vi "ResultsDB Create Barcode Items.vi"(6 "Order":T2, 8 "error in (no error)":errorcluster, 9 "File format":T1=".tdms", 10 "StationName":string, 11 "MainBarcode":string) -> (0 "error out":errorcluster, 2 "ResultFilePath":path, 3 "Row Numbers":string)   [LabVIEW 2021, in "SQLite.lvclass"]
doc: "开始测试时根据条目自动创建条目条目，生产文件路径。\n#2020-6-8 13:25:45"
uses:
  SQLite.lvclass
  Order.ctl
  File Format.ctl
  <vilib>/Utility/error.llb/Trim Whitespace.vi
  SQLite.lvclass/SQLite.ctl
  <userlib>/LabSQL/LabSQL.lvlib
  <userlib>/sushu/sushu.lvlib
  vi.lib_New/TopPath/TopPath.lvlib
panel:
  in  "error in (no error) 2":errorcluster
  out "CMD":string
  out "error out 2":errorcluster
  out "source":string
  out "match substring":string
  out "number (0 to 1)":dbl
  # "SQLITE_CONSTRAINT: UNIQUE constraint failed"
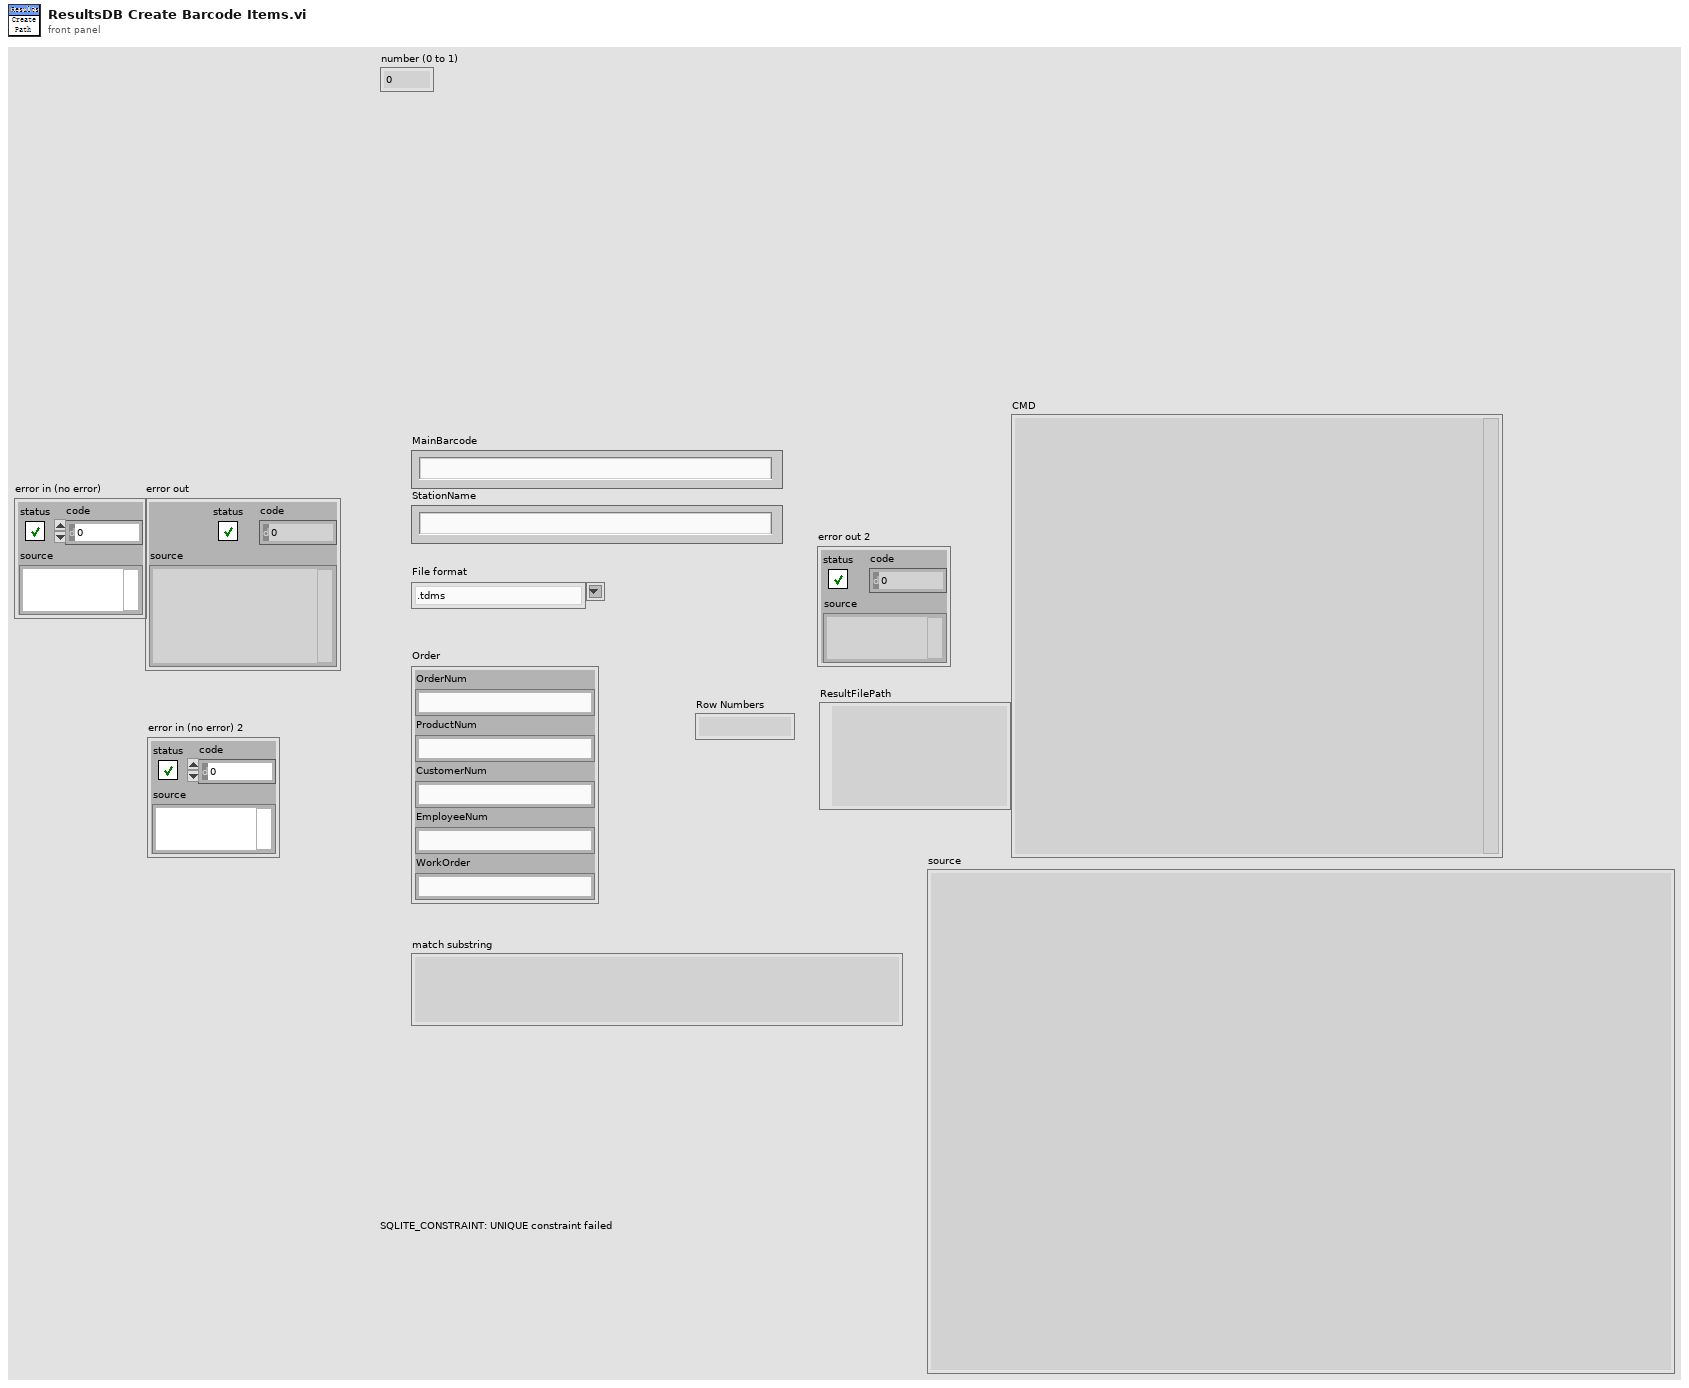
[diagram p1: front panel]
types:
  T1 = typedef "SQLite.lvclass/File Format.ctl" = string
  T2 = typedef "SQLite.lvclass/Order.ctl" = cluster{"OrderNum":string, "ProductNum":string, "CustomerNum":string, "EmployeeNum":string, "WorkOrder":string}
  T3 = cluster{"Core":cluster{"Current VI Reference":refnum<vi>, "Close Panel on Exit?":bool}, "VI Name":string, "Row Numbers":string, "Update?":bool, "Results Folder path":path, "CMD":string, "RowNum":i32, "ResultFilePath":path, "InsertTimes":i32}
  T4 = enum16{"Other", "SQL2008", "SQLite", "Access", "MySQL"}
  T5 = typedef "TopPath.lvlib/Top Path.ctl" = cluster{"LV Source":path, "FilePath":path, "Data":path}
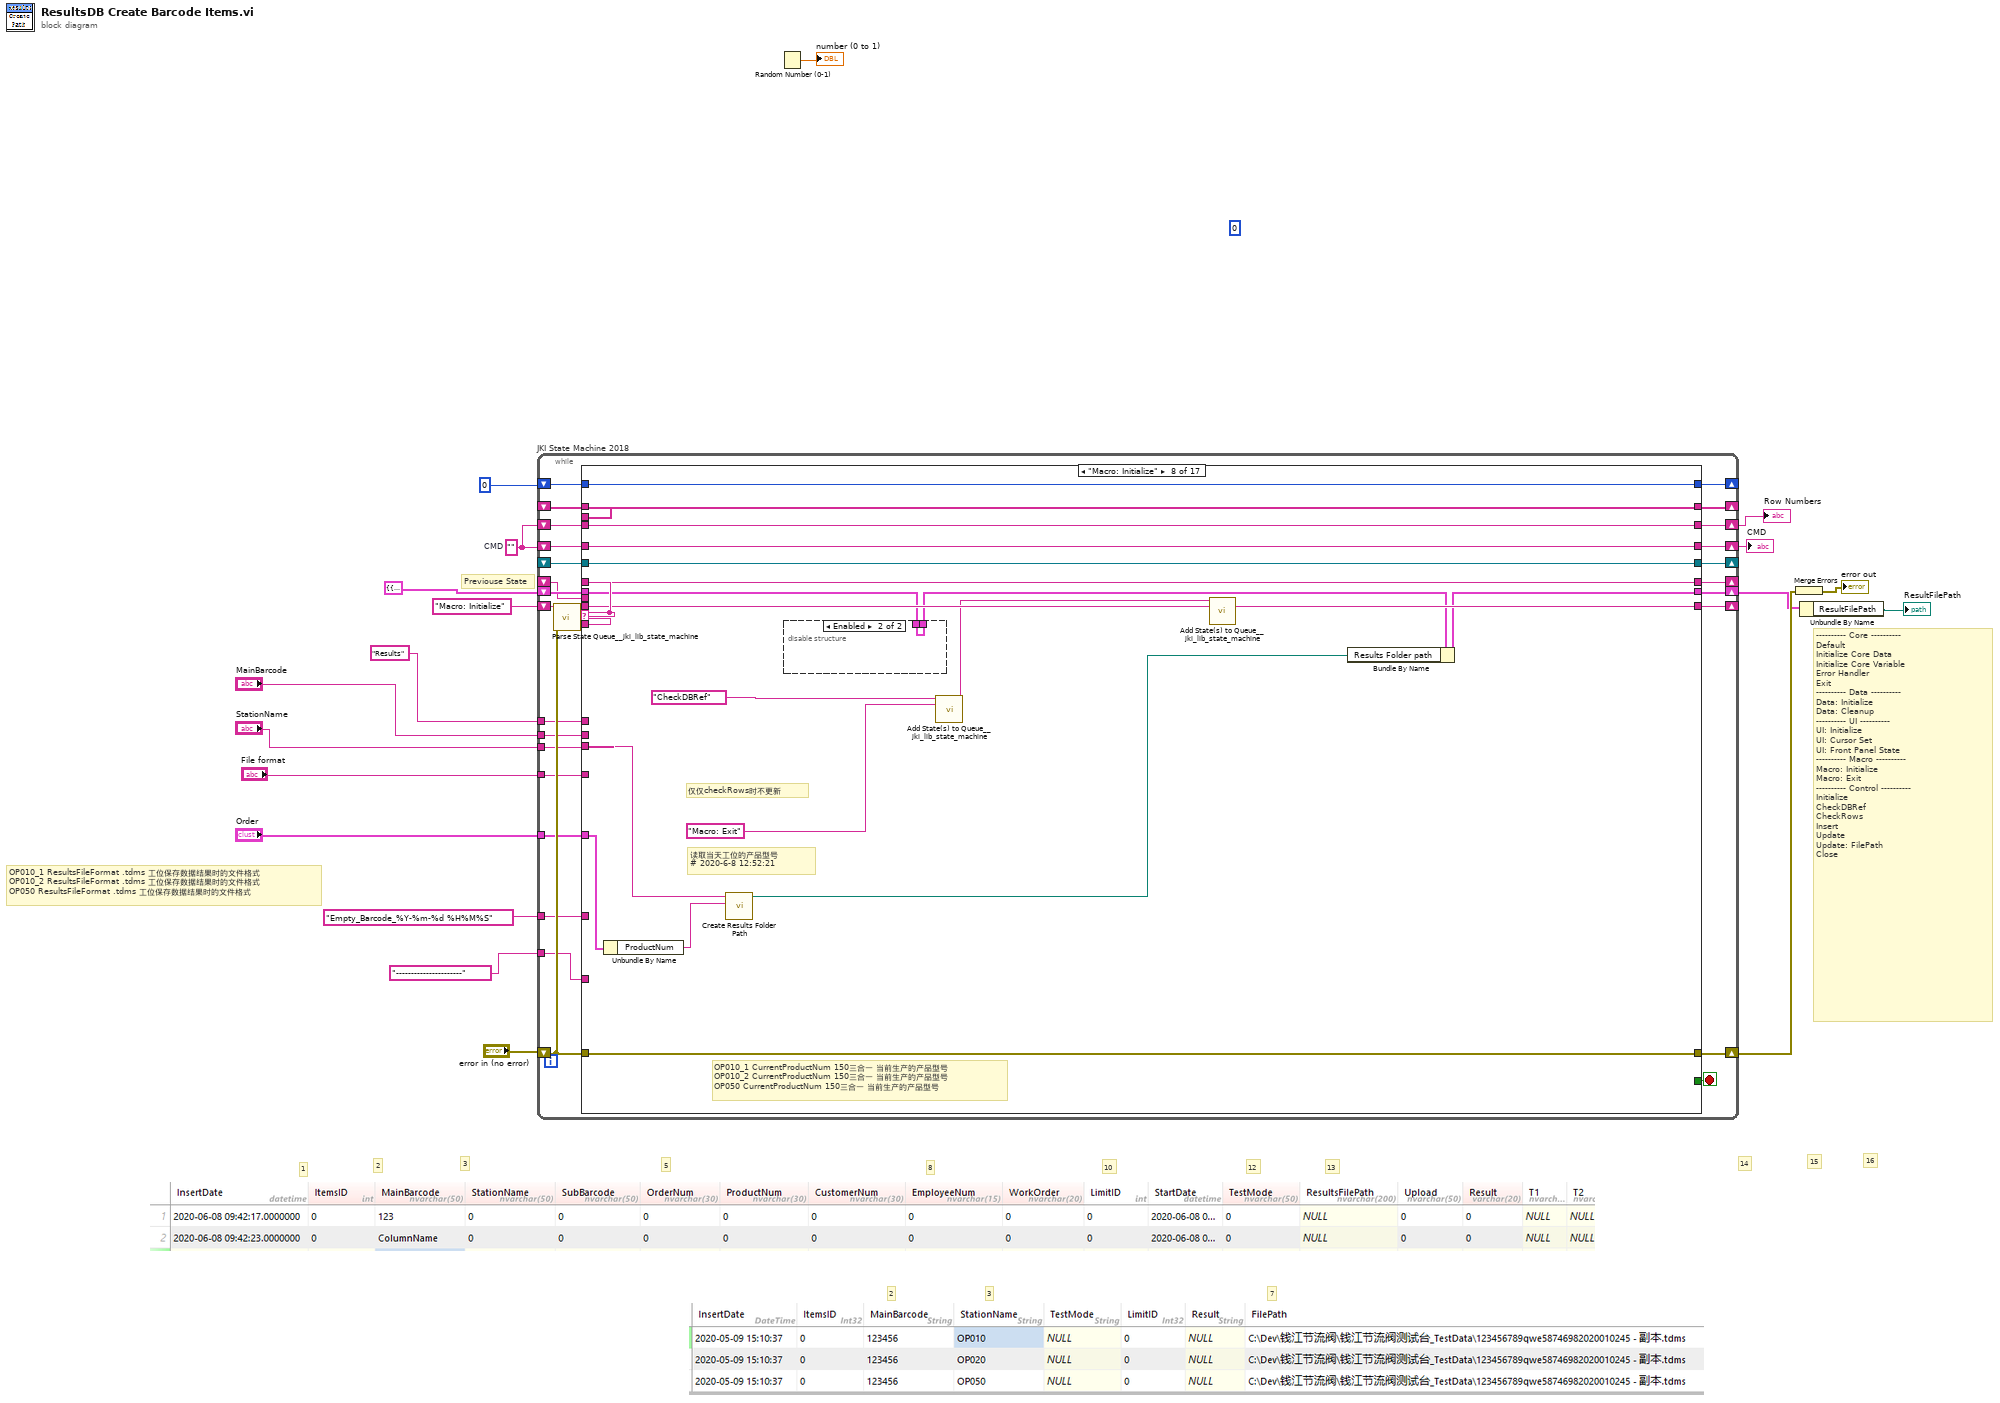
[diagram p0: block diagram]
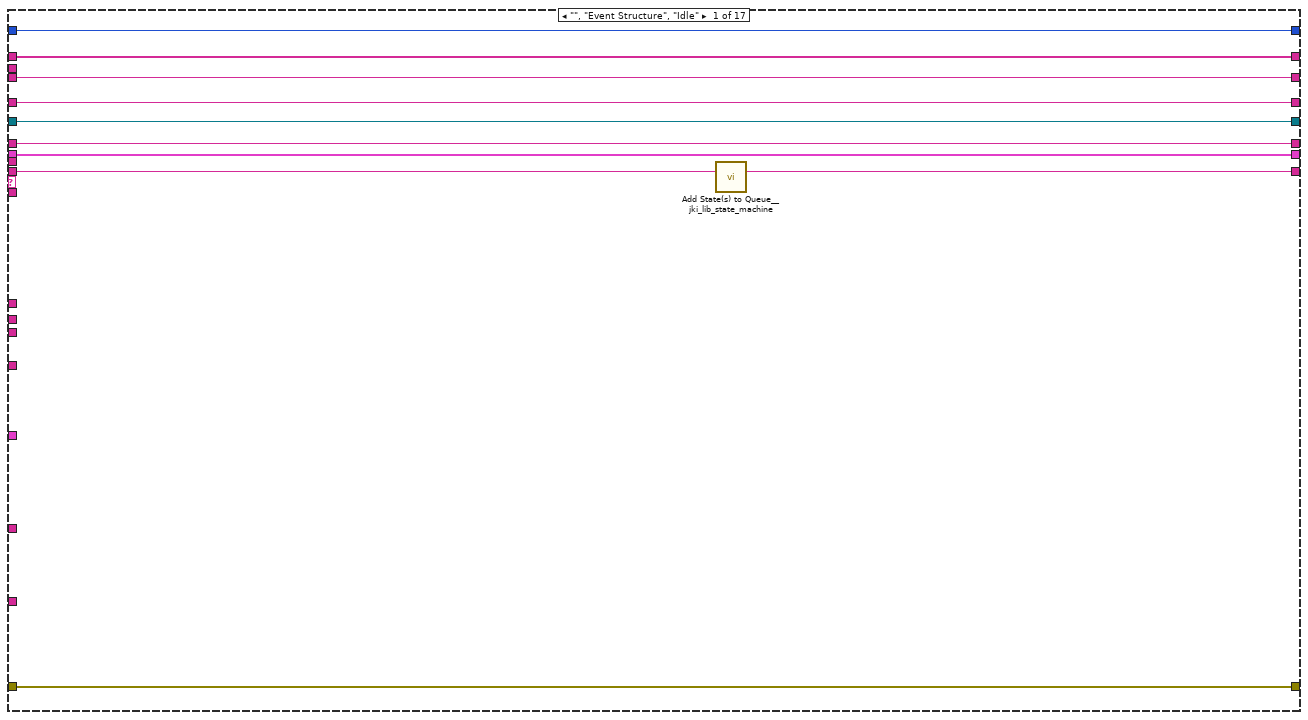
[diagram p2: hidden frame]
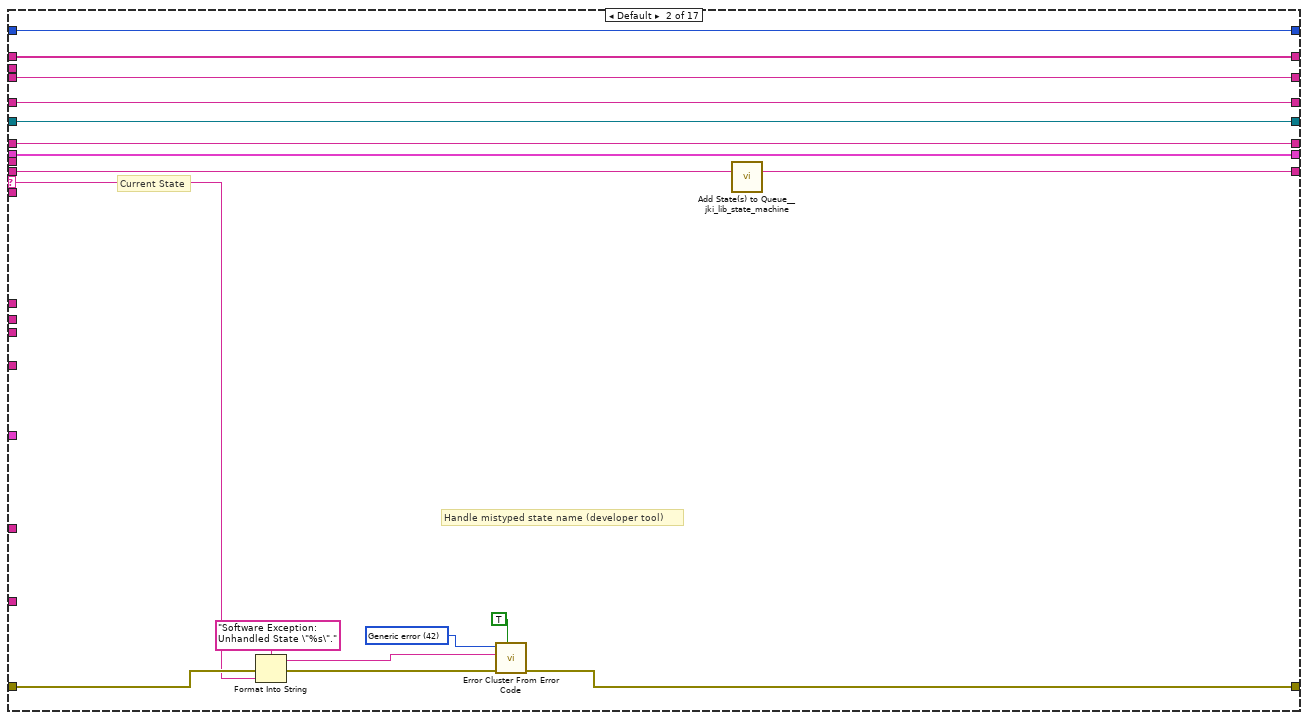
[diagram p3: hidden frame]
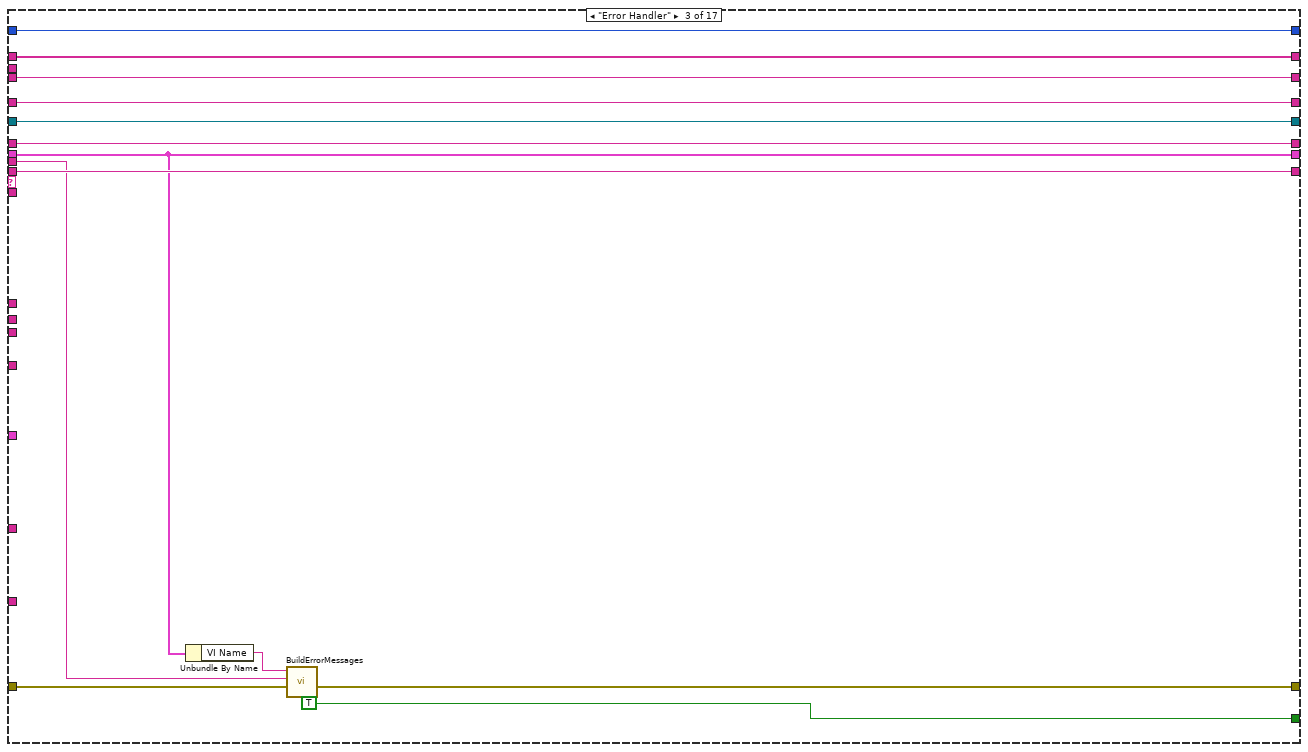
[diagram p4: hidden frame]
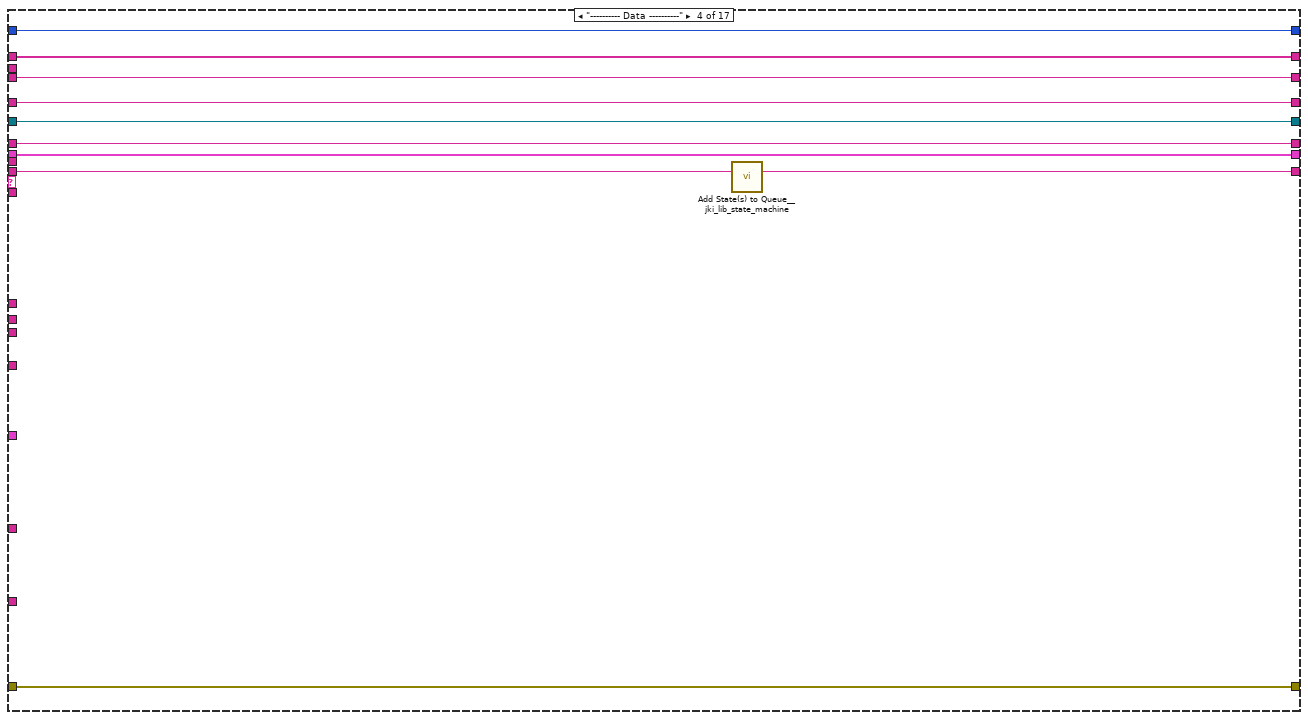
[diagram p5: hidden frame]
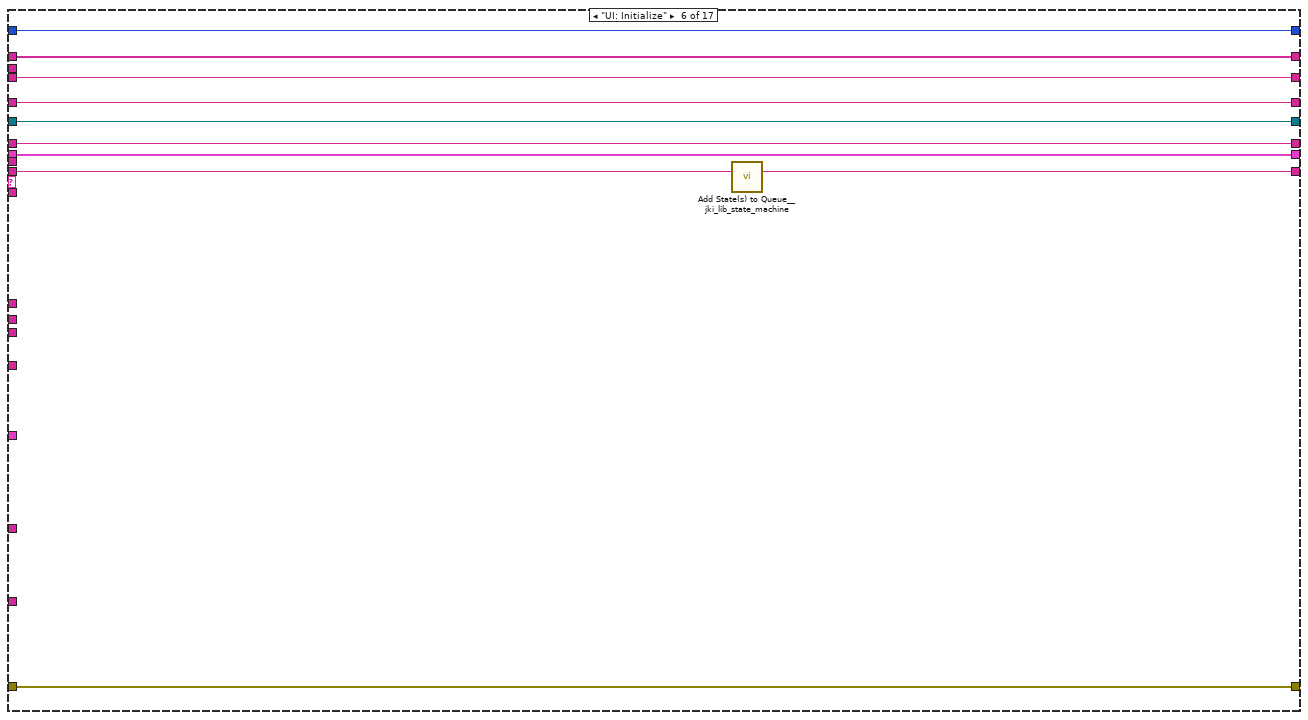
[diagram p7: hidden frame]
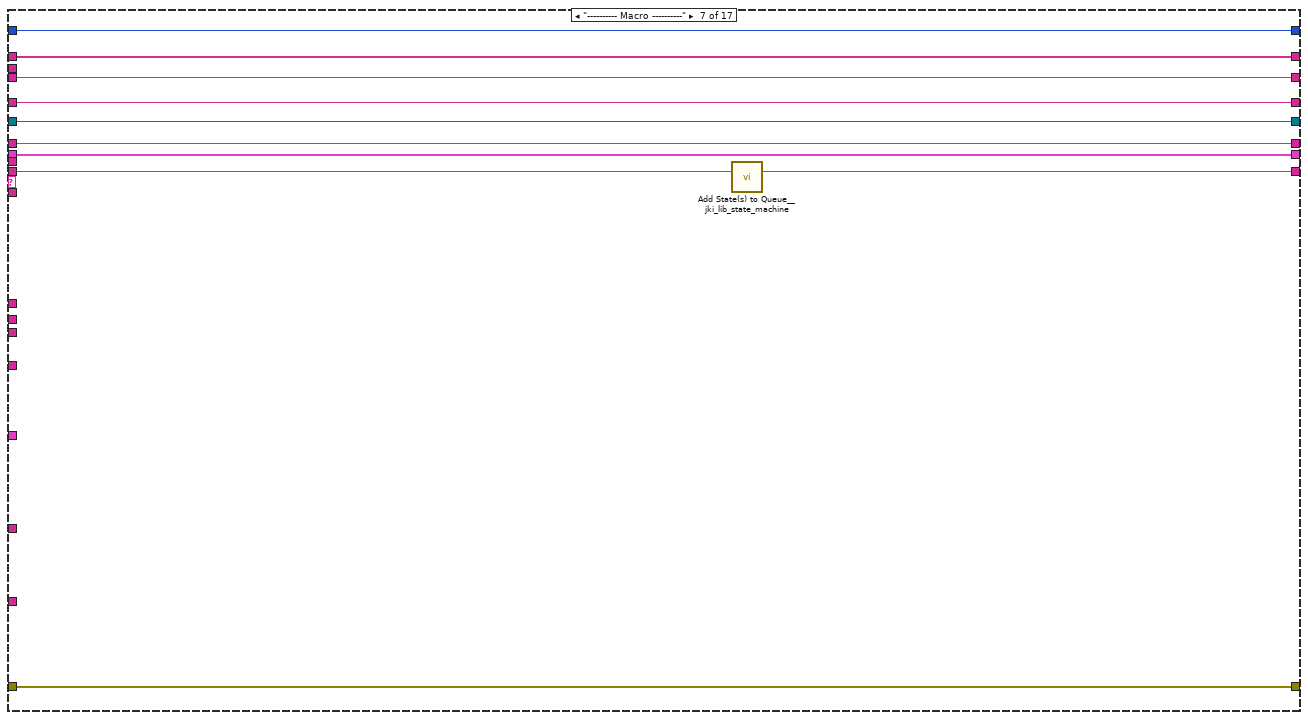
[diagram p8: hidden frame]
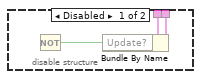
[diagram p9: hidden frame]
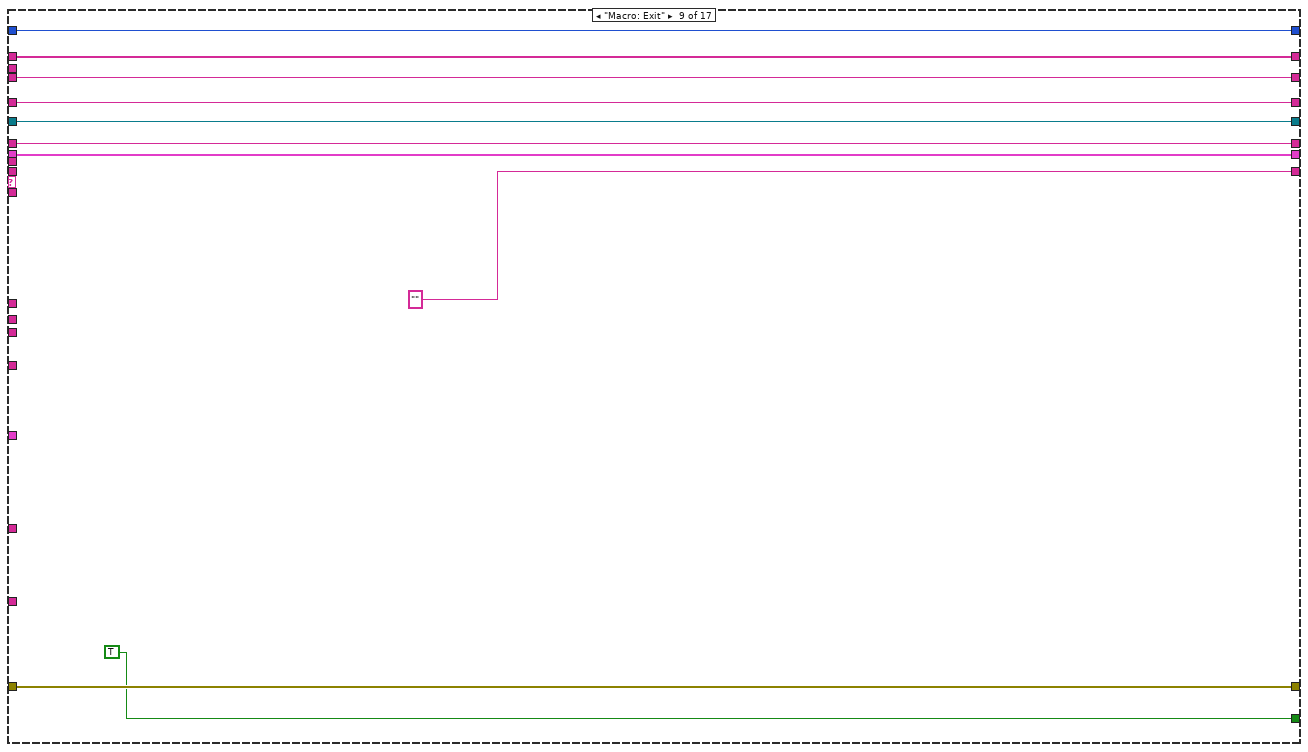
[diagram p10: hidden frame]
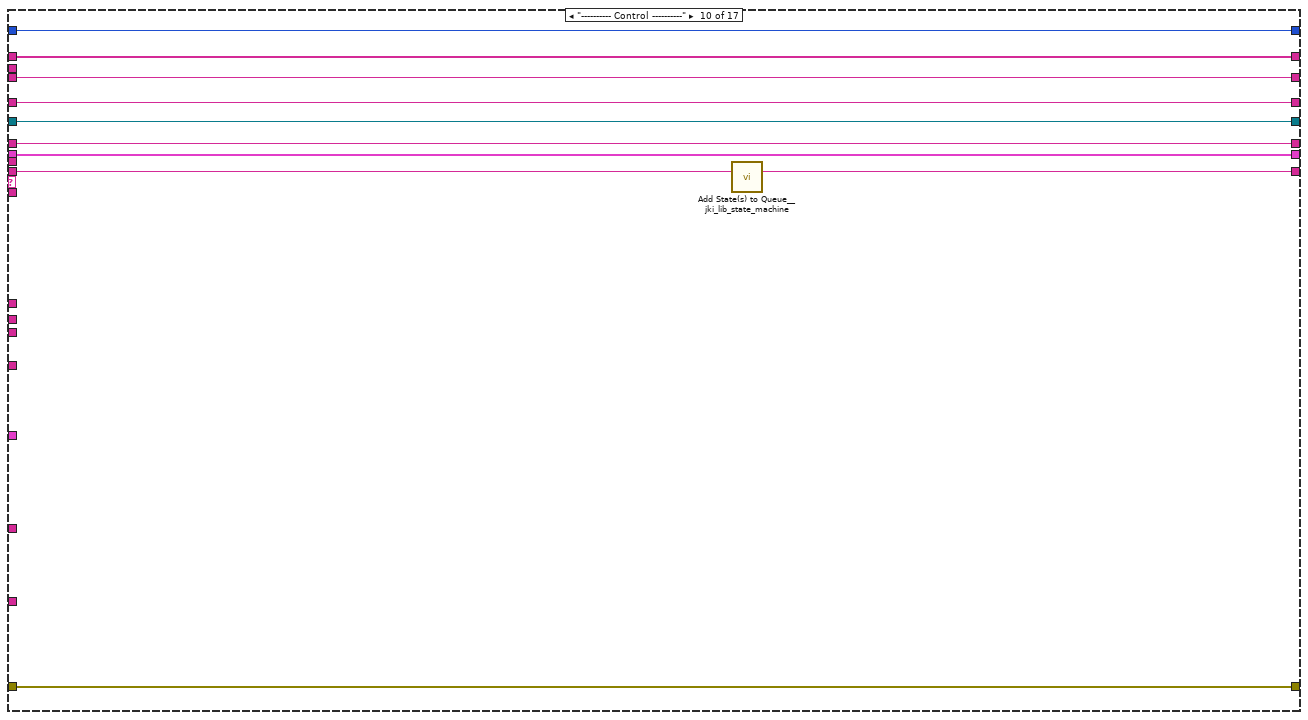
[diagram p11: hidden frame]
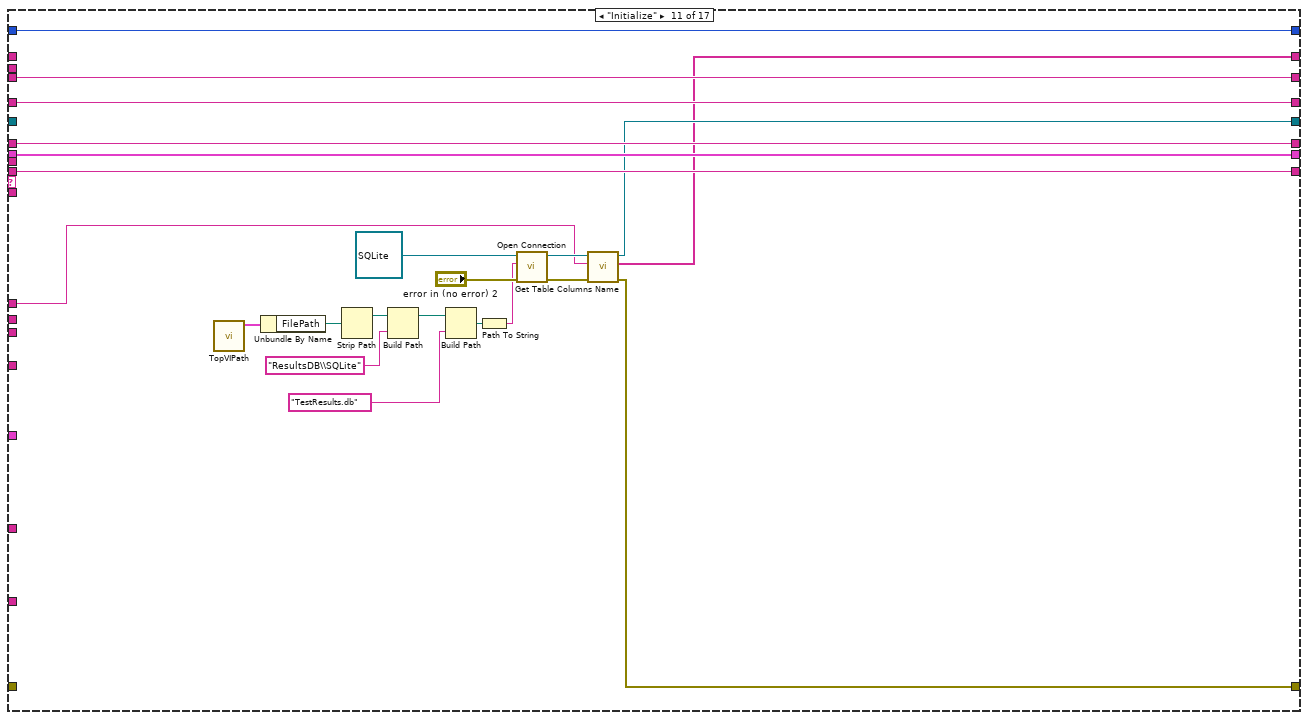
[diagram p12: hidden frame]
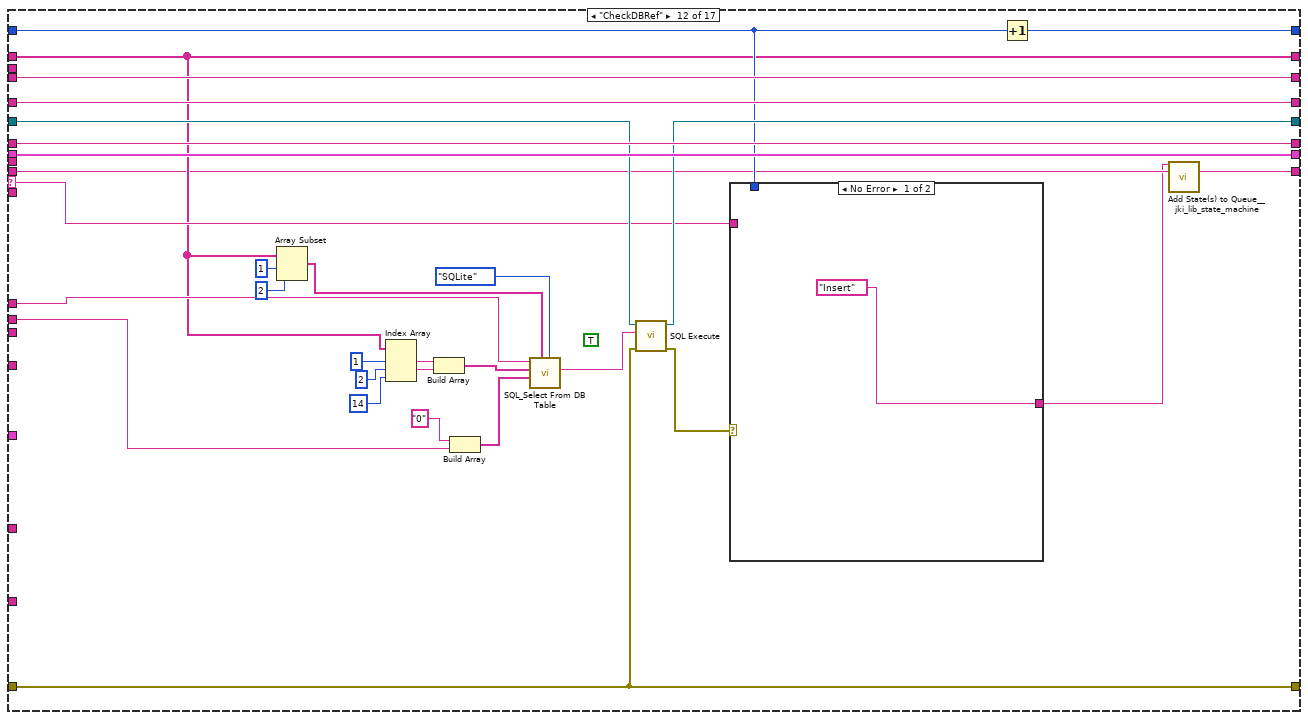
[diagram p13: hidden frame]
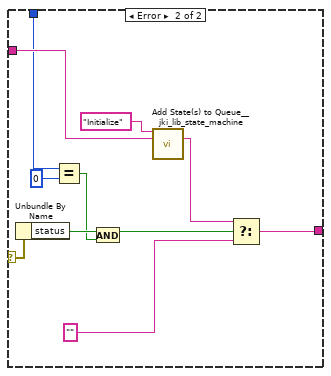
[diagram p14: hidden frame]
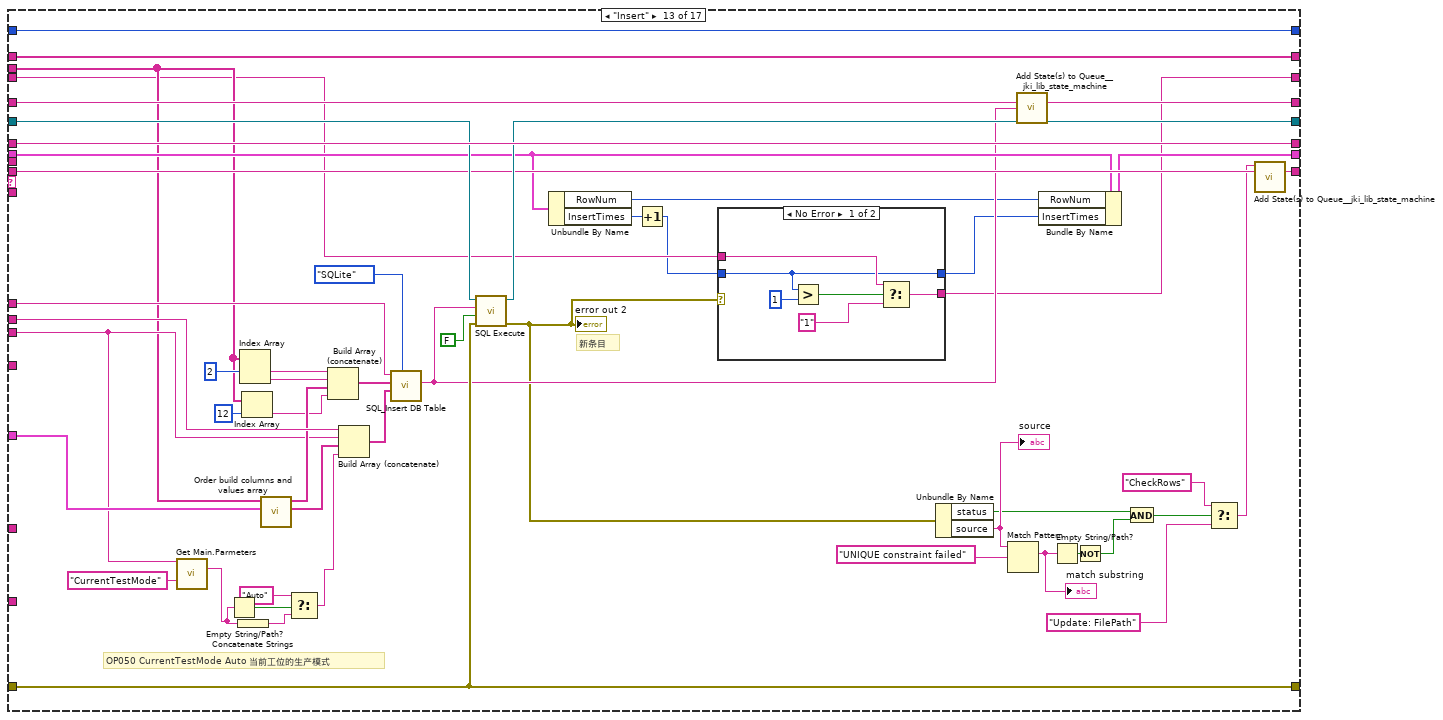
[diagram p15: hidden frame]
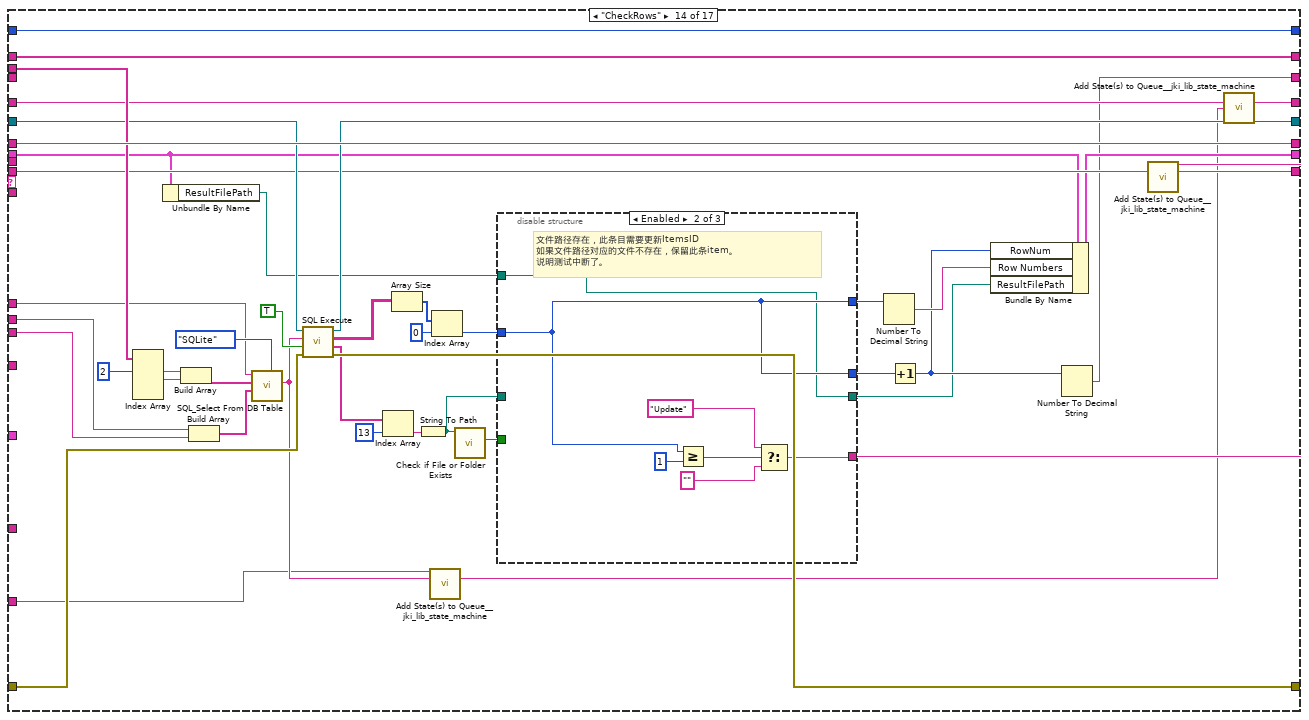
[diagram p17: hidden frame]
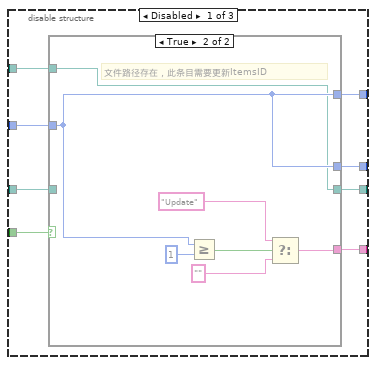
[diagram p18: hidden frame]
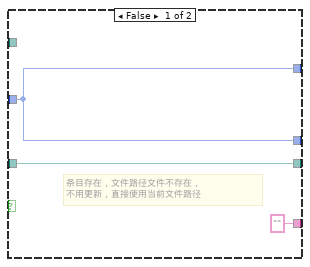
[diagram p19: hidden frame]
diagram:
  w4 = ""  # CMD
  (unwired) 0 ("index (row)")
  # "OP010_1\tResultsFileFormat\t.tdms\t工位保存数据结果时的文件格式\nOP010_2\tResultsFileFormat\t.tdms\t工位保存数据结果时的文件格式\nOP050\tResultsFileFormat\t.tdms\t工位保存数据结果时的文件格式"
  # "16"
  # "15"
  # "14"
  # "13"
  # "12"
  # "10"
  # "8"
  # "5"
  # "3"
  # "2"
  # "1"
  # "Previouse State"
  # "---------- Core ----------\nDefault\nInitialize Core Data\nInitialize Core Variable\nError Handler\nExit\n---------- Data ----------\nData: Initialize\nData: Cleanup\n---------- UI ----------\nUI: Initialize\nUI: Cursor Set\nUI: Front Panel State\n---------- Macro ----------\nMacro: Initialize\nMacro: Exit\n---------- Control ----------\nInitialize\nCheckDBRef\nCheckRows\nInsert\nUpdate\nUpdate: FilePath\nClose"
  # "7"
  # "3"
  # "2"
  n1 = while "JKI State Machine 2018" {
    shift-right: [w42] -> w7
    shift-left: T3 {"Core"={"Current VI Reference"=refnum, "Close Panel on Exit?"=FALSE}, "VI Name"="", "Row Numbers"="", "Update?"=FALSE, "Results Folder path"=path "", "CMD"="", "RowNum"=0, "ResultFilePath"=path "", "InsertTimes"=0} ("Data") -> [w41]
    shift-right: [w45] -> w15
    shift-left: "error in (no error)" -> [w40]
    shift-right: [w44] -> _
    shift-left: "Macro: Initialize" -> [w46]
    shift-right: [w38] -> _
    shift-left: _ -> [w39]
    shift-right: [w36] -> _
    shift-left: _ -> [w35]
    tunnel: "StationName" -> [w34]
    tunnel: "MainBarcode" -> [w33]
    tunnel: "Results" ("TableName") -> [w32]
    tunnel: "Order" -> [w31]
    tunnel: "File format" -> [w30]
    tunnel: "Empty_Barcode_%Y-%m-%d %H%M%S" ("time format string (%c)") -> [w29]
    shift-right: [w28] -> w8
    shift-left: w4 -> [w27]
    tunnel: "----------------------" ("State(s) in (\"\")") -> [w26]
    shift-right: [w24] -> w5
    shift-left: w4 -> [w25]
    shift-right: [w23] -> _
    shift-left: _ -> [w20]
    shift-right: [w21] -> _
    shift-left: 0 ("y") -> [w22]
    stop <- w43 stop-if-true
    n2 = call <vilib>:"Parse State Queue__jki_lib_state_machine.vi"("State Queue"=w46, "Error In (no error)"=w40) -> ("Remaining States"=w48:string, "Current State"=w37:string, "Arguments"=w47:string)  [unwired: 10 in, 1 out]
    n3 = case shown="\"Macro: Initialize\"" w37 {
      selector: w37 -> [_ w65 _ _ _ _ _ _ _ _ _ w205 _ _ _ _ _]
      tunnel: w48 -> [w58 w69 w87 w98 w104 w117 w127 w146 _ w170 w192 w194 w264 w323 w390 w453 w479]
      tunnel: w47 -> [_ _ _ _ _ _ _ _ _ _ _ _ _ _ _ _ _]
      tunnel: w41 -> [w55 w67 w84 w95 w105 w115 w124 w141 w159 w167 w191 w222 w258 w318 w389 w433 w478]
      tunnel: [w56 w71 w80 w96 w107 w114 w125 w142 w160 w168 w171 w209 w274 w321 w392 w418 w472] -> w45
      tunnel: w40 -> [w56 w70 w81 w96 w107 w114 w125 w142 w160 w168 _ w209 w274 w322 w392 w419 w473]
      tunnel: [w57 w68 w87 w97 w104 w116 w126 w145 "" w169 w192 w195 w265 w324 w391 w454 w479] -> w44
      tunnel: [_ _ TRUE _ _ _ _ _ TRUE _ _ _ _ _ _ _ _] -> w43
      tunnel: [w55 w67 w84 w95 w105 w115 w124 w136 w159 w167 w191 w222 w257 w319 w389 w426 w478] -> w42
      tunnel: w39 -> [w54 w64 w86 w94 w106 w113 w123 w144 w158 w166 _ w208 w277 w327 w395 w456 w474]
      tunnel: [w54 w64 w86 w94 w106 w113 w123 w144 w158 w166 w175 w207 w276 w326 w394 w455 w474] -> w38
      tunnel: w37 -> [w53 w63 w85 w93 w103 w112 w122 w143 w156 w165 w190 w221 w286 w338 w402 w461 w477]
      tunnel: [w53 w63 w85 w93 w103 w112 w122 w143 w156 w165 w190 w221 w286 w338 w402 w461 w477] -> w36
      tunnel: w35 -> [_ _ w82 _ _ _ _ _ _ _ _ _ _ _ _ _ _]
      tunnel: w34 -> [_ _ _ _ _ _ _ w133 _ _ _ _ w252 w328 w396 w423 _]
      tunnel: w33 -> [_ _ _ _ _ _ _ _ _ _ _ w202 w278 w329 w397 w414 _]
      tunnel: w20 -> [_ _ _ _ _ _ _ _ _ _ _ _ w250 w331 w384 w449 _]
      tunnel: w32 -> [_ _ _ _ _ _ _ _ _ _ w173 w206 w279 w330 w398 w457 _]
      tunnel: w31 -> [_ _ _ _ _ _ _ w129 _ _ _ _ w261 _ _ _ _]
      tunnel: w30 -> [_ _ _ _ _ _ _ _ _ _ _ _ _ _ _ w407 _]
      tunnel: w29 -> [_ _ _ _ _ _ _ _ _ _ _ _ _ _ _ w435 _]
      tunnel: w27 -> [w52 w62 w79 w92 w102 w111 w121 w135 w154 w164 w189 w220 w256 w316 w370 w431 w476]
      tunnel: [w52 w62 w79 w92 w102 w111 w121 w135 w154 w164 w189 w220 w255 w317 w371 w432 w476] -> w28
      tunnel: w26 -> [_ _ _ _ _ _ _ _ _ _ _ _ _ w313 w367 w428 _]
      tunnel: w25 -> [w51 w61 w78 w91 w101 w110 w120 w134 w153 w163 w188 w219 w246 _ w366 w417 w475]
      tunnel: [w51 w61 w78 w91 w101 w110 w120 w134 w153 w163 w188 w219 w245 w297 w366 w417 w475] -> w24
      tunnel: w20 -> [w49 w59 w76 w89 w99 w108 w118 w130 w151 w161 _ w199 w240 w295 w364 w415 w470]
      tunnel: [w49 w59 w76 w89 w99 w108 w118 w130 w151 w161 w172 w199 w240 w295 w364 w415 w470] -> w23
      tunnel: w22 -> [w50 w60 w77 w90 w100 w109 w119 w131 w152 w162 w174 w204 w241 w296 w365 w416 w471]
      tunnel: [w50 w60 w77 w90 w100 w109 w119 w131 w152 w162 w174 w203 w241 w296 w365 w416 w471] -> w21
      frame "", "Event Structure", "Idle" {
        n4 = call <vilib>:"Add State(s) to Queue__jki_lib_state_machine.vi"("State(s) in (\"\")"=w58) -> ("States Out"=w57:string)  [unwired: 14 in]
      }
      frame Default {
        w74 = 42 items=["No error", "Argument error", "Memory is full", "Out of zone", "End of file", "File already open", "Generic file I/O error", "File not found", "File permission error", "Disk is full", "Duplicate path", "Too many files open", "System feature not enabled", "Resource file not found", "Cannot add resource", "Resource not found", "Image not found", "Image memory error", "Pen does not exist", "Config type invalid", "Config token not found", "Config parse error", "Config memory error", "Bad external code format", "Bad external code offset", "External code not present", "Null window", "Destroy window error", "Null menu", "Print aborted", "Bad print record", "Print driver error", "Windows error during printing", "Memory error during printing", "Print dialog error", "Generic print error", "Invalid device refnum", "Device not found", "Device parameter error", "Device unit error", "Cannot open device", "Device call aborted", "Generic error", "Cancelled by user", "Object ID too low", "Object ID too high", "Object not in heap", "Unknown heap", "Unknown object (invalid DefProc)", "Unknown object (DefProc not in table)", "Message out of range", "Invalid (null) method", "Unknown message", "Manager call not supported", "Bad address", "Network operation in progress", "Network operation timed out", "Connection is busy", "Network attribute not supported", "Network error", "Address in use", "System out of memory", "Connection aborted", "Connection refused", "Not connected", "Already connected", "Connection closed", "Initialization error (interapplication manager)", "Bad occurrence", "Wait on unbound occurrence handler", "Occurrence queue overflow", "Datalog type conflict", "Unused", "Unrecognized type (interapplication manager)", "Memory corrupt", "Failed to make temporary DLL", "Old CIN version", "Drag socket not found", "Failed to load drop-object", "Failed to register OLE object", "Failed to release OLE object", "Format specifier type mismatch", "Unknown format specifier", "Too few format specifiers", "Too many format specifiers", "Scan failed", "Newer CIN version", "Error converting to variant", "Runtime menu error", "Password tampered", "Variant attribute not found", "Incompatible variant data type", "Event data is not available", "Event Store is not present", "Occurrence is not found", "Event Queue is not created", "Event info is not available", "Refnum passed is NULL", "Error retrieving Class GUID", "Error retrieving CoClass GUID", "Error retrieving TypeLib GUID.", "Bad built application magic bytes.", "Specific driver is different from the specific driver associated with the Logical Name.", "There is no session opened to the class driver.", "Max Error", "MAX - Error with config objects", "MAX - Error loading configuration", "MAX - Group not supported"]
        # "Current State"
        # "Handle mistyped state name (developer tool)"
        n5 = Format Into String(format string="Software Exception: Unhandled State \"%s\"." ("message"), error in=w70, w65) -> (resulting string=w73:string, error out=w72:errorcluster)  [unwired: 1 in]
        n6 = call <vilib>:"Error Cluster From Error Code.vi"("show call chain? (False)"=TRUE, "error in (no error)"=w72, "error message (\"\")"=w73, "error code (0)"=w74) -> ("error out"=w71:errorcluster)  [unwired: 5 in]
        n7 = call <vilib>:"Add State(s) to Queue__jki_lib_state_machine.vi"("State(s) in (\"\")"=w69) -> ("States Out"=w68:string)  [unwired: 14 in]
      }
      frame "Error Handler" {
        n8 = Unbundle By Name(w84) -> ("VI Name"=w83:string)
        n9 = call <userlib>:"BuildErrorMessages.vi"("error in"=w81, "ErrorCase"=w82, "VI Name"=w83) -> ("error out (no error)"=w80:errorcluster)  [unwired: 6 in, 2 out]
      }
      frame "---------- Data ----------" {
        n10 = call <vilib>:"Add State(s) to Queue__jki_lib_state_machine.vi"("State(s) in (\"\")"=w98) -> ("States Out"=w97:string)  [unwired: 14 in]
      }
      frame "Data: Initialize" {
      }
      frame "UI: Initialize" {
        n11 = call <vilib>:"Add State(s) to Queue__jki_lib_state_machine.vi"("State(s) in (\"\")"=w117) -> ("States Out"=w116:string)  [unwired: 14 in]
      }
      frame "---------- Macro ----------" {
        n12 = call <vilib>:"Add State(s) to Queue__jki_lib_state_machine.vi"("State(s) in (\"\")"=w127) -> ("States Out"=w126:string)  [unwired: 14 in]
      }
      frame "Macro: Initialize" {
        # "读取当天工位的产品型号\n# 2020-6-8 12:52:21"
        # "OP010_1\tCurrentProductNum\t150三合一\t当前生产的产品型号\nOP010_2\tCurrentProductNum\t150三合一\t当前生产的产品型号\nOP050\tCurrentProductNum\t150三合一\t当前生产的产品型号"
        # "仅仅checkRows时不更新"
        n13 = Unbundle By Name(w129) -> ("ProductNum"=w128:string)
        n14 = call "Create Results Folder Path.vi"("CurrentProductNum"=w128, "StationName"=w133) -> ("Folder path"=w132:path)  [unwired: 9 in]
        n15 = disable-structure shown="Enabled" {
          disable-tunnel: w141 -> [w149 w150]
          disable-tunnel: [w148 w150] -> w138
          frame Disabled {
            n16 = Not() -> (.not. x?=w147:bool)  [unwired: 1 in]
            n17 = Bundle By Name(cluster=w149, "Update?"=w147) -> (w148:T3)
          }
          frame Enabled {
          }
        }
        n18 = call <vilib>:"Add State(s) to Queue__jki_lib_state_machine.vi"("State(s) in Front (\"\")"="CheckDBRef" ("CMD"), "State(s) in (\"\")"="Macro: Exit") -> ("States Out"=w140:string)  [unwired: 13 in]
        n19 = call <vilib>:"Add State(s) to Queue__jki_lib_state_machine.vi"("State(s) in Front (\"\")"=w140, "State(s) in (\"\")"=w146) -> ("States Out"=w145:string)  [unwired: 13 in]
        n20 = Bundle By Name(cluster=w138, "Results Folder path"=w132) -> (w136:T3)
      }
      frame "Macro: Exit" {
      }
      frame "---------- Control ----------" {
        n21 = call <vilib>:"Add State(s) to Queue__jki_lib_state_machine.vi"("State(s) in (\"\")"=w170) -> ("States Out"=w169:string)  [unwired: 14 in]
      }
      frame "Initialize" {
        n22 = call "TopVIPath.vi"() -> ("TopPath"=w187:T5)  [unwired: 10 in, 1 out]
        n23 = Unbundle By Name(w187) -> ("FilePath"=w176:path)
        n24 = Strip Path(path=w176) -> (stripped path=w177:path)  [unwired: 1 out]
        n25 = Build Path(base path=w177, name or relative path="ResultsDB\\SQLite") -> (appended path=w179:path)
        n26 = Build Path(base path=w179, name or relative path="TestResults.db") -> (appended path=w181:path)
        n27 = Path To String(path=w181) -> (string=w182:string)
        n28 = call-dynamic "Open Connection.vi"("error in (no error)"="error in (no error) 2", "ConnectionString"=w182, "HostDB in"=refnum<class "SQLite.lvclass"> refnum ("SQLite.lvclass")) -> ("error out"=w185:errorcluster, "HostDB out"=w184:refnum<class "SQLite.lvclass">)  [unwired: 7 in]
        n29 = call-dynamic "Get Table Columns Name.vi"("error in (no error)"=w185, "TableName"=w173, "HostDB in"=w184) -> ("error out"=w171:errorcluster, "Table_ColunmsList"=w172:string[], "HostDB out"=w175:refnum<class "SQLite.lvclass">)  [unwired: 4 in, 2 out]
      }
      frame "CheckDBRef" {
        (unwired) TRUE ("Return Data (T)")
        n30 = Array Subset(array=w199, index=1, length=2) -> (w196:string[])
        n31 = Index Array(array=w199, index #1=1 ("index"), index #2=2 ("index"), index #3=14 ("index")) -> (element #1=w201:string, element #2=w212:string)  [unwired: 1 out]
        n32 = Build Array(w201, w212) -> (w217:string[])
        n33 = Build Array("0" ("element"), w202) -> (w216:string[])
        n34 = call <userlib>:"SQL_Select From DB Table.vi"("DB Type"=T4."SQLite", "SelectedColumnsNameList"=w196, "ColumnsValue"=w216, "ColumnsNameList"=w217, "TableName"=w206) -> ("Select SQL CMD"=w214:string)  [unwired: 6 in]
        n35 = call-dynamic "SQL Execute.vi"("error in (no error)"=w209, "Command Text"=w214, "HostDB in"=w208) -> ("error out"=w210:errorcluster, "HostDB out"=w207:refnum<class "SQLite.lvclass">)  [unwired: 4 in, 3 out]
        n36 = case shown="No Error" w210 {
          selector: w210 -> [_ w230]
          tunnel: w205 -> [_ w231]
          tunnel: ["Insert" ("CMD") w229] -> w193
          tunnel: w204 -> [_ w226]
          frame No Error {
          }
          frame Error {
            n37 = Unbundle By Name(w230) -> ("status"=w228:bool)
            n38 = Equal?(x=w226, y=0) -> (x = y?=w224:bool)
            n39 = And(x=w228, y=w224) -> (x .and. y?=w227:bool)
            n40 = call <vilib>:"Add State(s) to Queue__jki_lib_state_machine.vi"("State(s) in Front (\"\")"="Initialize" ("Remaining States"), "State(s) in (\"\")"=w231) -> ("States Out"=w232:string)  [unwired: 13 in]
            n41 = Select(t=w232, s=w227, f="") -> (s? t:f=w229:string)
          }
        }
        n42 = Increment(x=w204) -> (x+1=w203:i32)
        n43 = call <vilib>:"Add State(s) to Queue__jki_lib_state_machine.vi"("State(s) in Front (\"\")"=w193, "State(s) in (\"\")"=w194) -> ("States Out"=w195:string)  [unwired: 13 in]
      }
      frame "Insert" {
        # "OP050\tCurrentTestMode\tAuto\t当前工位的生产模式"
        # "新条目"
        n44 = call "Get Main.Parmeters.vi"("Main"=w252, "VariableName"="CurrentTestMode") -> ("Value"=w236:string)  [unwired: 6 in, 7 out]
        n45 = Empty String/Path?(string/path=w236) -> (empty?=w239:bool)
        n46 = Concatenate Strings(w236) -> (w238:string)
        n47 = Index Array(array=w250, index #1=2 ("index")) -> (element #1=w284:string, element #2=w285:string)  [unwired: 1 in]
        n48 = Index Array(array=w250, index=12) -> (element=w248:string)
        n49 = call "Order build columns and values array.vi"("Order"=w261, "ColunmsList"=w250) -> ("Order values Array"=w259:string[], "Order Columns Array"=w260:string[])  [unwired: 8 in]
        n50 = Select(t="Auto", s=w239, f=w238) -> (s? t:f=w235:string)
        n51 = Build Array (concatenate)(w284, w285, w260, w248) -> (w282:string[])
        n52 = Build Array (concatenate)(w278, w252, w259, w235) -> (w281:string[])
        n53 = call <userlib>:"SQL_Insert DB Table.vi"("DB Type"=T4."SQLite", "ColumnsValue"=w281, "ColumnsName"=w282, "Table Name"=w279) -> ("Insert DB String"=w254:string)  [unwired: 7 in]
        n54 = call-dynamic "SQL Execute.vi"("error in (no error)"=w274, "Return Data (T)"=FALSE, "Command Text"=w254, "HostDB in"=w277) -> ("error out"=w247:errorcluster, "HostDB out"=w276:refnum<class "SQLite.lvclass">)  [unwired: 3 in, 3 out]
        "error out 2" <- w247
        n55 = Unbundle By Name(w258) -> ("RowNum"=w253:i32, "InsertTimes"=w243:i32)
        n56 = Increment(x=w243) -> (x+1=w242:i32)
        n57 = case shown="No Error" w247 {
          tunnel: w242 -> [w287 w293]
          tunnel: w246 -> [w290 w294]
          tunnel: [w289 w294] -> w245
          tunnel: [w287 w293] -> w244
          frame No Error {
            n58 = Greater?(x=w287, y=1) -> (0:w291:bool)
            n59 = Select(t=w290, s=w291, f="1") -> (s? t:f=w289:string)
          }
          frame Error {
          }
        }
        n60 = Unbundle By Name(w247) -> ("status"=w270:bool, "source"=w273:string)
        "source" <- w273
        n61 = Match Pattern(string=w273, regular expression="UNIQUE constraint failed") -> (match substring=w271:string)  [unwired: 1 in, 3 out]
        "match substring" <- w271
        n62 = call <vilib>:"Add State(s) to Queue__jki_lib_state_machine.vi"("State(s) in (\"\")"=w256, "State(s) at Back (\"\")"=w254) -> ("States Out"=w255:string)  [unwired: 13 in]
        n63 = Bundle By Name(cluster=w258, "RowNum"=w253, "InsertTimes"=w244) -> (w257:T3)
        n64 = Empty String/Path?(string/path=w271) -> (empty?=w269:bool)
        n65 = Not(x=w269) -> (.not. x?=w262:bool)
        n66 = And(x=w270, y=w262) -> (x .and. y?=w268:bool)
        n67 = Select(t="CheckRows", s=w268, f="Update: FilePath") -> (s? t:f=w263:string)
        n68 = call <vilib>:"Add State(s) to Queue__jki_lib_state_machine.vi"("State(s) in Front (\"\")"=w263, "State(s) in (\"\")"=w264) -> ("States Out"=w265:string)  [unwired: 13 in]
      }
      frame "CheckRows" {
        n69 = Index Array(array=w331, index #1=2 ("index")) -> (element #1=w336:string, element #2=w337:string)  [unwired: 3 in, 2 out]
        n70 = Unbundle By Name(w318) -> ("ResultFilePath"=w298:path)
        n71 = Build Array(w336, w337) -> (w334:string[])
        n72 = Build Array(w329, w328) -> (w333:string[])
        n73 = call <userlib>:"SQL_Select From DB Table.vi"("DB Type"=T4."SQLite", "ColumnsValue"=w333, "ColumnsNameList"=w334, "TableName"=w330) -> ("Select SQL CMD"=w314:string)  [unwired: 7 in]
        n74 = call-dynamic "SQL Execute.vi"("error in (no error)"=w322, "Return Data (T)"=TRUE, "Command Text"=w314, "HostDB in"=w327) -> ("error out"=w321:errorcluster, "FirstRow"=w309:string[], "Table Control"=w303:string[][], "HostDB out"=w326:refnum<class "SQLite.lvclass">)  [unwired: 3 in, 1 out]
        n75 = Index Array(array=w309, index=13) -> (element=w307:string)
        n76 = Array Size(array=w303) -> (size(s)=w304:i32[])
        n77 = String To Path(string=w307) -> (path=w299:path)
        n78 = call <vilib>:"Add State(s) to Queue__jki_lib_state_machine.vi"("State(s) in Front (\"\")"=w313, "State(s) in (\"\")"=w314) -> ("States Out"=w315:string)  [unwired: 13 in]
        n79 = Index Array(array=w304, index=0) -> (element=w302:i32)
        n80 = call <vilib>:"Check if File or Folder Exists.vi"("path"=w299) -> ("file or folder exists?"=w306:bool)  [unwired: 8 in, 2 out]
        n81 = disable-structure shown="Enabled" {
          disable-tunnel: [w346 w363 _] -> w320
          disable-tunnel: [w345 w362 _] -> w311
          disable-tunnel: w306 -> [w344 _ _]
          disable-tunnel: w302 -> [w343 w362 _]
          disable-tunnel: [w342 w362 _] -> w301
          disable-tunnel: [w341 w361 _] -> w300
          disable-tunnel: w299 -> [w340 _ _]
          disable-tunnel: w298 -> [w339 w361 _]
          frame Disabled {
            n82 = case shown="True" w344 {
              tunnel: ["" ("f") w354] -> w346
              tunnel: [w348 w351] -> w345
              tunnel: w343 -> [w348 w351]
              tunnel: [w348 w351] -> w342
              tunnel: [w347 w350] -> w341
              tunnel: w340 -> [w347 _]
              tunnel: w339 -> [_ w350]
              frame False {
                # "条目存在，文件路径文件不存在，\n不用更新，直接使用当前文件路径"
              }
              frame True {
                # "文件路径存在，此条目需要更新ItemsID"
                n83 = Greater Or Equal?(x=w351, y=1) -> (x >= y?=w352:bool)
                n84 = Select(t="Update", s=w352, f="") -> (s? t:f=w354:string)
              }
            }
          }
          frame Enabled {
            # "文件路径存在，此条目需要更新ItemsID\n如果文件路径对应的文件不存在，保留此条item。\n说明测试中断了。"
            n85 = Greater Or Equal?(x=w362, y=1) -> (x >= y?=w357:bool)
            n86 = Select(t="Update", s=w357, f="") -> (s? t:f=w363:string)
          }
          frame Disabled {
          }
        }
        n87 = Number To Decimal String(number=w311) -> (decimal integer string=w312:string)  [unwired: 1 in]
        n88 = Increment(x=w301) -> (x+1=w310:i32)
        n89 = Bundle By Name(cluster=w318, "RowNum"=w310, "Row Numbers"=w312, "ResultFilePath"=w300) -> (w319:T3)
        n90 = Number To Decimal String(number=w310) -> (decimal integer string=w297:string)  [unwired: 1 in]
        n91 = call <vilib>:"Add State(s) to Queue__jki_lib_state_machine.vi"("State(s) in Front (\"\")"=w320, "State(s) in (\"\")"=w323) -> ("States Out"=w324:string)  [unwired: 13 in]
        n92 = call <vilib>:"Add State(s) to Queue__jki_lib_state_machine.vi"("State(s) in (\"\")"=w316, "State(s) at Back (\"\")"=w315) -> ("States Out"=w317:string)  [unwired: 13 in]
      }
      frame "Update" {
        n93 = Unbundle By Name(w389) -> ("Row Numbers"=w388:string)
        n94 = Index Array(array=w384, index=1) -> (element=w401:string)
        n95 = Index Array(array=w384, index #1=1 ("index")) -> (element #1=w383:string, element #2=w382:string, element #3=w381:string)  [unwired: 2 in]
        n96 = Build Array("0" ("element"), w397, w396) -> (w378:string[])
        n97 = Build Array(w383, w382, w381) -> (w380:string[])
        n98 = Build Array(w401) -> (w399:string[])
        n99 = Build Array(w388) -> (w387:string[])
        n100 = call <userlib>:"Build string_ColumnsName=ColumnsValue_Where and.vi"("DB Type"=T4."SQLite", "ColumnsValue"=w378, "Check ASCII?"=FALSE, "ColumnsNameList"=w380) -> ("ColumnName='ColumnValue'"=w386:string)  [unwired: 7 in]
        n101 = call <userlib>:"SQL_Update DB Table.vi"("where name='value'"=w386, "ColumnsValue"=w387, "ColumnsNameList"=w399, "TableName"=w398) -> ("Update CMD"=w368:string)  [unwired: 7 in]
        n102 = call-dynamic "SQL Execute.vi"("error in (no error)"=w392, "Return Data (T)"=FALSE, "Command Text"=w368, "HostDB in"=w395) -> ("error out"=w375:errorcluster, "HostDB out"=w394:refnum<class "SQLite.lvclass">)  [unwired: 3 in, 3 out]
        n103 = Select(t="", s=w375, f="Insert") -> (s? t:f=w373:string)
        n104 = call <vilib>:"Add State(s) to Queue__jki_lib_state_machine.vi"("State(s) in Front (\"\")"=w367, "State(s) in (\"\")"=w368) -> ("States Out"=w369:string)  [unwired: 13 in]
        n105 = call <vilib>:"Add State(s) to Queue__jki_lib_state_machine.vi"("State(s) in Front (\"\")"=w373, "State(s) in (\"\")"=w390) -> ("States Out"=w391:string)  [unwired: 13 in]
        n106 = call <vilib>:"Add State(s) to Queue__jki_lib_state_machine.vi"("State(s) in (\"\")"=w370, "State(s) at Back (\"\")"=w369) -> ("States Out"=w371:string)  [unwired: 13 in]
      }
      frame "Update: FilePath" {
        w412 = "_" ("string")
        # "0\t测试产品编号\t1"
        # "写文件路径到数据库。# 2020-6-8 15:49:02"
        # "OP010_1\tResultsFileFullPath\tC:\\Dev\\钱江节流阀\\ResultsData\\2020-06-08\\OP050\\150三合一\\1234.tdms\nOP010_2\tResultsFileFullPath\tC:\\Dev\\钱江节流阀\\ResultsData\\2020-06-08\\OP050\\150三合一\\1234.tdms\nOP050\tResultsFileFullPath\tC:\\Dev\\钱江节流阀\\ResultsData\\2020-06-08\\OP050\\150三合一\\1234.tdms"
        n107 = Unbundle By Name(w433) -> ("Results Folder path"=w434:path, "RowNum"=w427:i32)  [unwired: 1 out]
        n108 = call "Replace Backslash.vi"("Barcode"=w414) -> ("连接的字符串"=w410:string)  [unwired: 10 in]
        n109 = call "Get Main.Parmeters.vi"("VariableName"="测试产品编号") -> ("Value"=w411:string)  [unwired: 7 in, 7 out]
        n110 = Concatenate Strings(w410, w412, w411) -> (w409:string)
        n111 = case shown="2.." w427 {
          selector: w427 -> [_ w465 _]
          tunnel: w409 -> [w462 w467 w469]
          tunnel: [w462 w466 w468] -> w436
          tunnel: w412 -> [_ w463 _]
          frame Default {
          }
          frame 2.. {
            n112 = Number To Decimal String(number=w465) -> (decimal integer string=w464:string)  [unwired: 1 in]
            n113 = Concatenate Strings(w467, w463, w464) -> (w466:string)
          }
          frame 0 {
            n114 = Concatenate Strings(w469) -> (w468:string)
          }
        }
        n115 = call "Get Main.Parmeters.vi"("Main"=w423, "VariableName"="ResultsFileFormat") -> ("Value"=w406:string)  [unwired: 6 in, 7 out]
        n116 = Concatenate Strings(w407) -> (w403:string)
        n117 = Empty String/Path?(string/path=w406) -> (empty?=w408:bool)
        n118 = Concatenate Strings(w406) -> (w404:string)
        n119 = Empty String/Path?(string/path=w436) -> (empty?=w440:bool)
        n120 = Format Date/Time String(time format string (%c)=w435) -> (date/time string=w439:string)  [unwired: 2 in]
        n121 = Select(t=w403, s=w408, f=w404) -> (s? t:f=w405:string)
        n122 = Select(t=w439, s=w440, f=w436) -> (s? t:f=w437:string)
        n123 = Concatenate Strings(w437, w405) -> (w438:string)
        n124 = Build Path(base path=w434, name or relative path=w438) -> (appended path=w425:path)
        n125 = Path To String(path=w425) -> (string=w421:string)
        n126 = Index Array(array=w449, index=13) -> (element=w460:string)
        n127 = Index Array(array=w449, index #1=1 ("index")) -> (element #1=w448:string, element #2=w447:string, element #3=w446:string)  [unwired: 2 in]
        n128 = Build Array("0" ("element"), w414, w423) -> (w443:string[])
        n129 = Build Array(w448, w447, w446) -> (w445:string[])
        n130 = Build Array(w460) -> (w458:string[])
        n131 = Build Array(w421) -> (w452:string[])
        n132 = call <userlib>:"Build string_ColumnsName=ColumnsValue_Where and.vi"("DB Type"=T4."SQLite", "ColumnsValue"=w443, "Check ASCII?"=FALSE, "ColumnsNameList"=w445) -> ("ColumnName='ColumnValue'"=w451:string)  [unwired: 7 in]
        n133 = call <userlib>:"SQL_Update DB Table.vi"("where name='value'"=w451, "ColumnsValue"=w452, "ColumnsNameList"=w458, "TableName"=w457) -> ("Update CMD"=w429:string)  [unwired: 7 in]
        n134 = call-dynamic "SQL Execute.vi"("error in (no error)"=w419, "Command Text"=w429, "HostDB in"=w456) -> ("error out"=w420:errorcluster, "HostDB out"=w455:refnum<class "SQLite.lvclass">)  [unwired: 4 in, 3 out]
        n135 = call <vilib>:"Add State(s) to Queue__jki_lib_state_machine.vi"("State(s) in Front (\"\")"=w428, "State(s) in (\"\")"=w429) -> ("States Out"=w430:string)  [unwired: 13 in]
        n136 = Bundle By Name(cluster=w433, "ResultFilePath"=w425) -> (w426:T3)
        n137 = call "Update Main.Parmeters.vi"("VariableName"="ResultsFileFullPath", "Main"=w423, "Value"=w421, "error in (no error)"=w420) -> ("error out"=w418:errorcluster)  [unwired: 11 in]
        n138 = call <vilib>:"Add State(s) to Queue__jki_lib_state_machine.vi"("State(s) in (\"\")"=w431, "State(s) at Back (\"\")"=w430) -> ("States Out"=w432:string)  [unwired: 13 in]
        n139 = call <vilib>:"Add State(s) to Queue__jki_lib_state_machine.vi"("State(s) in (\"\")"=w453) -> ("States Out"=w454:string)  [unwired: 14 in]
      }
      frame "Close" {
        n140 = call-dynamic "Close Connection.vi"("error in (no error)"=w473, "HostDB in"=w474) -> ("error out"=w472:errorcluster)  [unwired: 8 in, 1 out]
      }
    }
  }
  "CMD" <- w8
  "Row Numbers" <- w5
  n141 = Random Number (0-1)() -> (number: 0 to 1=→"number (0 to 1)":dbl)
  n142 = Merge Errors(w15) -> (→"error out":errorcluster)
  n143 = Unbundle By Name(w7) -> ("ResultFilePath"=→"ResultFilePath":path)
